vi "Calibration Filename (Read).vi"(6 "ISOBUS address":T2=-1 caption="ISOBUS address (-1)", 8 "error in":errorcluster, 11 "Mercury Reference In":T3) -> (0 "error out":errorcluster, 2 "Calibration Filename":string, 3 "Mercury Reference Out":T3, 4 "Valid?":T1)   [LabVIEW 2018, in "Mercury iXX.lvlib" / "Temperature.lvlib"]
doc: "Read the current calibration file for the selected temperature device."
uses:
  Temperature.lvlib
  Mercury Reference.ctl
  Comms Transport Layer.ctl
  Query Dynamic Reference.ctl
  ISOBus Address.ctl
  Is Valid LED.ctl
  Command Verbs.ctl
  Mercury iXX.lvlib
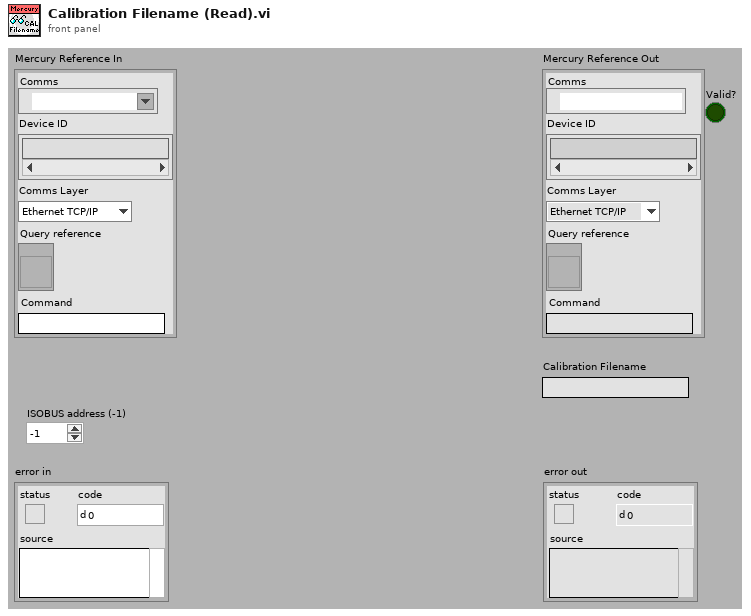
[diagram p1: front panel]
types:
  T1 = typedef "Mercury iXX.lvlib/Is Valid LED.ctl" = bool
  T2 = typedef "Mercury iXX.lvlib/ISOBus Address.ctl" = i32
  T3 = typedef "Mercury iXX.lvlib/Mercury Reference.ctl" = cluster{"Comms":refnum<visa-resource-name>, "Device ID":string[], "Comms Layer":T4, "Command":string, "Query reference":T5}
  T4 = typedef "Mercury iXX.lvlib/Comms Transport Layer.ctl" = enum16{"Ethernet TCP/IP", "USB", "ISOBus - RS-232", "GPIB"}
  T5 = typedef "Mercury iXX.lvlib/Query Dynamic Reference.ctl" = refnum<vi>
  T6 = typedef "Mercury iXX.lvlib/Command Verbs.ctl" = string
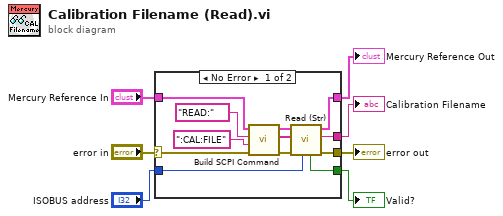
[diagram p0: block diagram]
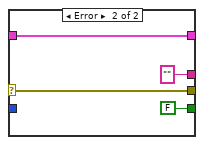
[diagram p2: hidden frame]
diagram:
  n1 = case shown="No Error" "error in" {
    selector: "error in" -> [w8 w23]
    tunnel: "Mercury Reference In" -> [w14 w22]
    tunnel: [w13 w22] -> w6
    tunnel: [w12 "" ("Response")] -> w5
    tunnel: [w11 w23] -> w4
    tunnel: [w10 T1 FALSE ("Valid?")] -> w3
    tunnel: "ISOBUS address" -> [w9 _]
    frame No Error {
      n2 = call "Build SCPI Command.vi"("error in"=w8, "Noun(s)"=":CAL:FILE" ("Command"), "Verb"=T6 "READ:", "Mercury Reference In"=w14) -> ("error out"=w19:errorcluster, "SCPI Message(s)"=w16:string[], "Mercury Reference Out"=w17:T3)  [unwired: 5 out]
      n3 = call "Read (Str).vi"("ISOBUS address"=w9, "error in"=w19, "SCPI Message(s)"=w16, "Mercury Reference In"=w17) -> ("error out"=w11:errorcluster, "Response"=w12:string, "Mercury Reference Out"=w13:T3, "Valid?"=w10:T1)  [unwired: 4 out]
    }
    frame Error {
    }
  }
  "Mercury Reference Out" <- w6
  "error out" <- w4
  "Calibration Filename" <- w5
  "Valid?" <- w3
